vi "NumberRows.vi"(8 "error in (no error)":errorcluster, 11 "Table Ref in":refnum<vi>) -> (0 "error out":errorcluster, 3 "Table Ref out":refnum<vi>)   [LabVIEW 2013]
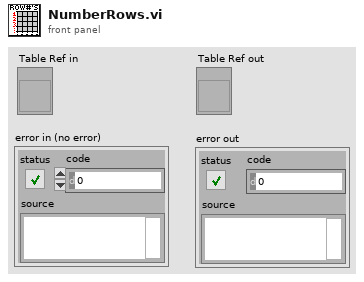
[diagram p1: front panel]
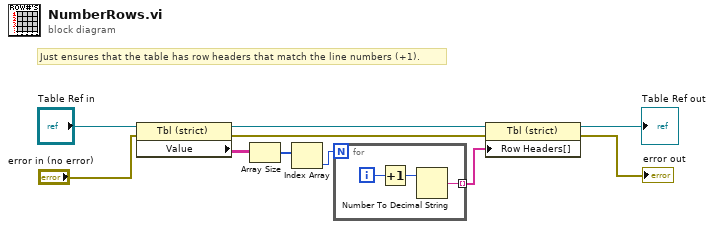
[diagram p0: block diagram]
diagram:
  # "Just ensures that the table has row headers that match the line numbers (+1)."
  n1 = property on="Property Node" class="Tbl (strict)"(reference="Table Ref in", error in="error in (no error)") -> (reference out=w4:refnum<vi>, error out=w2:errorcluster, "Value"=w6:string[][])
  n2 = Array Size(array=w6) -> (size(s)=w9:i32[])
  n3 = Index Array(array=w9) -> (element=w8:i32)  [unwired: 1 in]
  n4 = for {
    N: w8 -> [_]
    tunnel: [w11] -> w7 mode=indexing
    i -> [w13]
    n5 = Increment(x=w13) -> (x+1=w12:i32)
    n6 = Number To Decimal String(number=w12) -> (decimal integer string=w11:string)  [unwired: 1 in]
  }
  n7 = property on="Property Node" class="Tbl (strict)"(reference=w4, error in=w2, "Row Headers[]"=w7) -> (reference out=→"Table Ref out":refnum<vi>, error out=→"error out":errorcluster)
